vi "escritura_de_I1.vi"(0 "I1\n<0,0|0,0>":bool, 1 "String":string, 2 "Array":dbl[](array[numeric])) -> ()   [LabVIEW 2013]
uses:
  <vilib>/Utility/file.llb/Write To Spreadsheet File (string).vi
panel:
  in  "file path (dialog if empty)":path=path "C:/Users/franjas/Documents/rutinas-calibracion-slm/parametros_medida.txt"
  in  "ICImagingControl":refnum<k7>(container)
  in  "Array 2":string[][](array[string])=[["Pi", "Li", "Lo", "Po", "E", "B", "G", "C", "I1"], ["0", "0", "0", "0", "0", "48", "0", "0", "0"]]
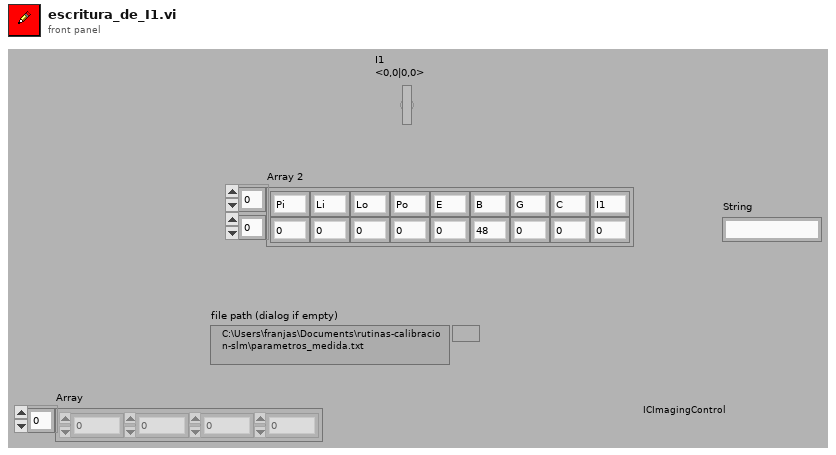
[diagram p1: front panel]
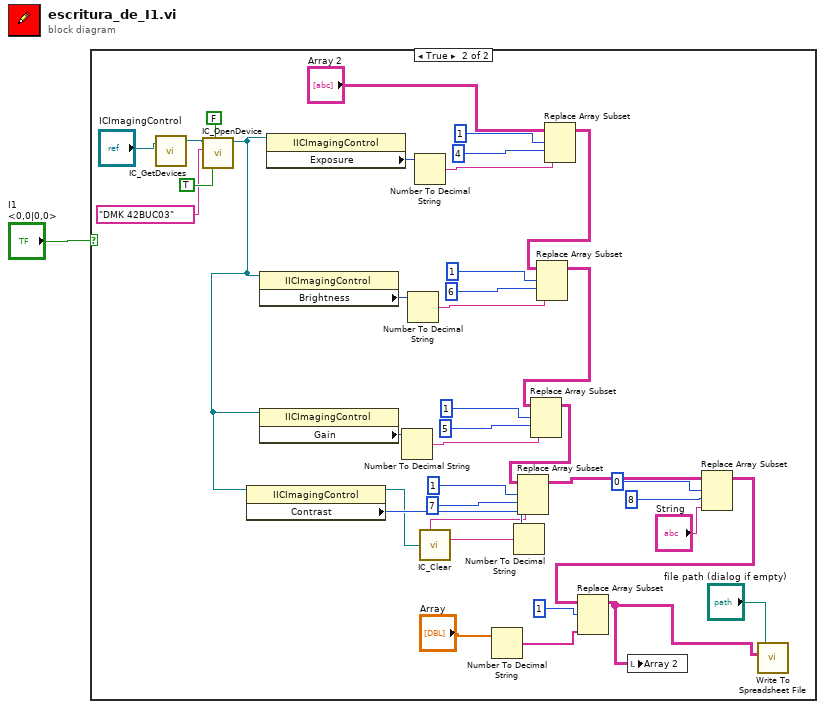
[diagram p0: block diagram]
diagram:
  n1 = case shown="True" "I1\n<0,0|0,0>" {
    frame False {
    }
    frame True {
      n2 = call <userlib>:"IC_GetDevices.vi"("ICImagingControl In"="ICImagingControl") -> ("ICImagingControl Out"=w37:refnum<k7>)  [unwired: 1 in, 2 out]
      n3 = call <userlib>:"IC_OpenDevice.vi"("Color"=FALSE, "Live"=TRUE, "Device"="DMK 42BUC03", "ICImagingControl In"=w37) -> ("ICImagingControl Out"=w14:refnum<k7>)  [unwired: 2 in, 5 out]
      n4 = property class="IICImagingControl"(reference=w14) -> (reference out=w11:refnum<k7>, "Contrast"=w18:i32)  [unwired: 1 in, 1 out]
      n5 = property class="IICImagingControl"(reference=w14) -> ("Brightness"=w30:i32)  [unwired: 1 in, 2 out]
      n6 = property class="IICImagingControl"(reference=w14) -> ("Gain"=w26:i32)  [unwired: 1 in, 2 out]
      n7 = property class="IICImagingControl"(reference=w14) -> ("Exposure"=w34:i32)  [unwired: 1 in, 2 out]
      n8 = Number To Decimal String(number=w26) -> (decimal integer string=w23:string)  [unwired: 1 in]
      n9 = Number To Decimal String(number=w30) -> (decimal integer string=w27:string)  [unwired: 1 in]
      n10 = Number To Decimal String(number=w34) -> (decimal integer string=w31:string)  [unwired: 1 in]
      n11 = call <userlib>:"IC_Clear.vi"("ICImagingControl 2"=w11) -> ()  [unwired: 1 out]
      n12 = Number To Decimal String(number="Array") -> (decimal integer string=w4:string[])  [unwired: 1 in]
      n13 = Number To Decimal String(number=w18) -> (decimal integer string=w15:string)  [unwired: 1 in]
      n14 = Replace Array Subset(array="Array 2", new element=w31, index (row)=1, index (col)=4 ("disabled index (col)")) -> (w20:string[][])
      n15 = Replace Array Subset(array=w20, new element=w27, index (row)=1, index (col)=6 ("disabled index (col)")) -> (w19:string[][])
      n16 = Replace Array Subset(array=w19, new element=w23, index (row)=1, index (col)=5 ("disabled index (col)")) -> (w13:string[][])
      n17 = Replace Array Subset(array=w13, new element=w15, index (row)=1, index (col)=7 ("disabled index (col)")) -> (w7:string[][])
      n18 = Replace Array Subset(array=w7, new element="String", index (row)=0, index (col)=8 ("disabled index (col)")) -> (w6:string[][])
      n19 = Replace Array Subset(array=w6, new element=w4, index (row)=1) -> (w2:string[][])  [unwired: 1 in]
      n20 = local write "Array 2"(w2) -> ()
      n21 = call-poly <vilib>:"Write To Spreadsheet File.vi"("2D data"=w2, "file path (dialog if empty)"="file path (dialog if empty)") -> ()  [unwired: 6 in, 1 out]
    }
  }
